vi "RTD_display_value.vi"(7 "type":T1=enum."COMET Tx5xx (ethernet)" caption="Type", 8 "error in":errorcluster, 9 "status code":i32, 10 "temp [deg C]":dbl, 11 "VISA in":refnum<visa-resource-name>) -> (0 "error out":errorcluster, 3 "VISA out":refnum<visa-resource-name>)   [LabVIEW 2020]
uses:
  thermo_types.ctl
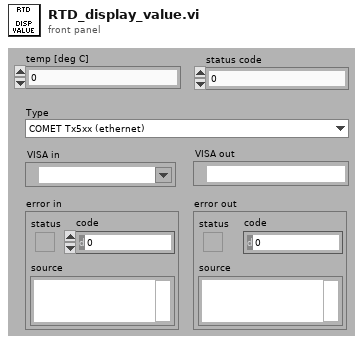
[diagram p1: front panel]
types:
  T1 = typedef "thermo_types.ctl" = enum16{"Disabled", "Simulated", "COMET Tx5xx (ethernet)", "Keithley 2002 (GPIB) + RTD", "Agilent 344xx (GPIB) + RTD"}
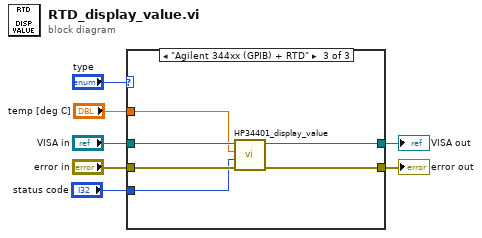
[diagram p0: block diagram]
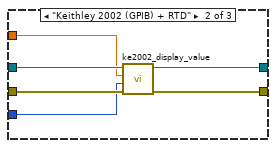
[diagram p3: hidden frame]
diagram:
  n1 = case shown="\"Agilent 344xx (GPIB) + RTD\"" "type" {
    tunnel: "error in" -> [w9 w15 w21]
    tunnel: [w9 w14 w20] -> w5
    tunnel: [w8 w13 w19] -> w4
    tunnel: "VISA in" -> [w8 w12 w18]
    tunnel: "temp [deg C]" -> [_ w11 w17]
    tunnel: "status code" -> [_ w10 w16]
    frame Default {
    }
    frame "Keithley 2002 (GPIB) + RTD" {
      n2 = call "ke2002_display_value.vi"("error in"=w15, "status code"=w10, "temp [deg C]"=w11, "VISA in"=w12) -> ("error out"=w14:errorcluster, "VISA out"=w13:refnum<visa-resource-name>)  [unwired: 6 in]
    }
    frame "Agilent 344xx (GPIB) + RTD" {
      n3 = call "HP34401_display_value.vi"("error in"=w21, "status code"=w16, "temp [deg C]"=w17, "VISA in"=w18) -> ("error out"=w20:errorcluster, "VISA out"=w19:refnum<visa-resource-name>)  [unwired: 6 in]
    }
  }
  "error out" <- w5
  "VISA out" <- w4
